vi "ziImpedanceCalibRefZ.vi"(3 "Frequencies (Hz)":dbl[](array[numeric]), 4 "Model Values":cdb[](array[numeric]), 5 "Eq Model (Unity)":T1) -> (0 "Z (Ohm)":cdb[](array[numeric]), 1 "cal_types":cluster{string[], bool[]}[](array[cluster]))   [LabVIEW 2016, in "Zurich Instruments LabOne.lvlib"]
doc: "Calculates the nominal impedance of the equivalent circuit model of the calibration reference for the frequencies used in the current measurement."
uses:
  Zurich Instruments LabOne.lvlib
  ziTypeImpedanceEqCircModel.ctl
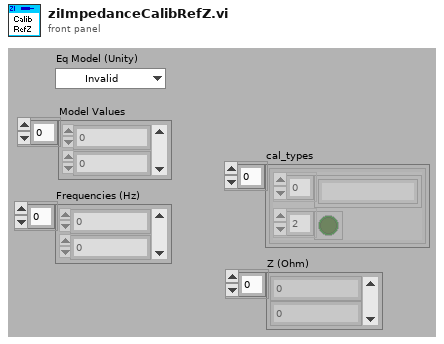
[diagram p1: front panel]
types:
  T1 = typedef "Zurich Instruments LabOne.lvlib/ziTypeImpedanceEqCircModel.ctl" = enum16{"Invalid", "|Z|, Phi", "R||C", "R||L", "R*C", "D*C", "R*L", "ReZ, ImZ", "G, B"}
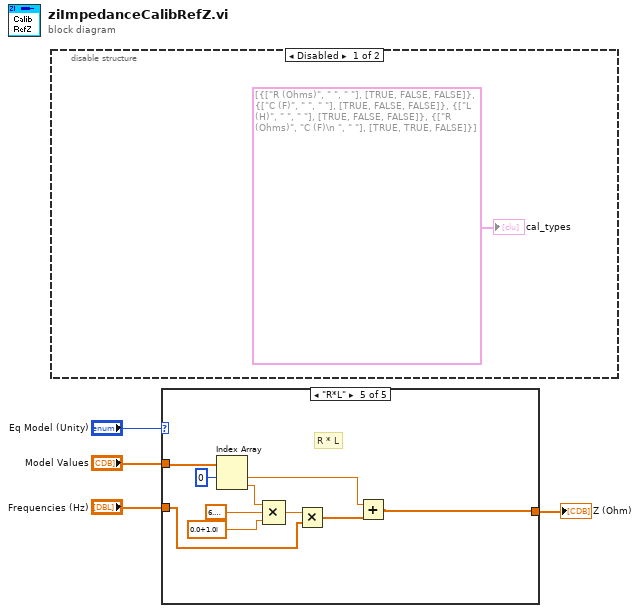
[diagram p0: block diagram]
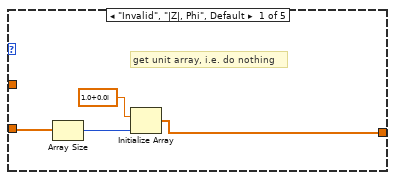
[diagram p3: hidden frame]
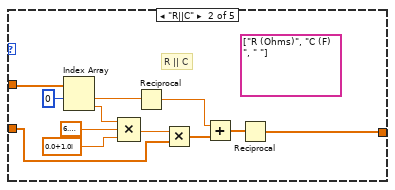
[diagram p4: hidden frame]
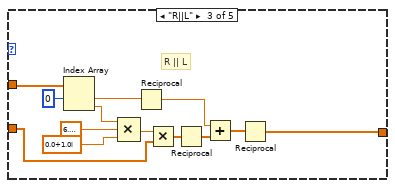
[diagram p5: hidden frame]
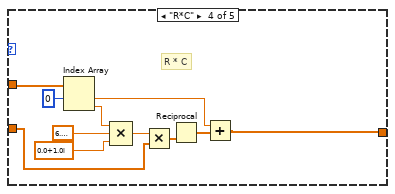
[diagram p6: hidden frame]
diagram:
  n1 = disable-structure shown="Disabled" {
    frame Disabled {
      "cal_types" <- cluster{string[], bool[]}[] [{["R (Ohms)", " ", " "], [TRUE, FALSE, FALSE]}, {["C (F)", " ", " "], [TRUE, FALSE, FALSE]}, {["L (H)", " ", " "], [TRUE, FALSE, FALSE]}, {["R (Ohms)", "C (F)\n ", " "], [TRUE, TRUE, FALSE]}]
    }
    frame Enabled {
    }
  }
  n2 = case shown="\"R*L\"" "Eq Model (Unity)" {
    tunnel: "Frequencies (Hz)" -> [w8 w11 w24 w35 w47]
    tunnel: [w6 w13 w26 w38 w49] -> w4
    tunnel: "Model Values" -> [_ w20 w33 w44 w54]
    frame "Invalid", "|Z|, Phi", Default {
      # "get unit array, i.e. do nothing"
      n3 = Array Size(array=w8) -> (size(s)=w9:i32)
      n4 = Initialize Array(cdb 1.0+0.0i, w9) -> (w6:cdb[])
    }
    frame "R||C" {
      (unwired) string[] ["R (Ohms)", "C (F) ", " "]
      # "R || C"
      n5 = Index Array(array=w20, index #1=0 ("index")) -> (element #1=w16:cdb, element #2=w17:cdb)  [unwired: 1 in]
      n6 = Compound Arithmetic op=MULTIPLY(w17, 6.283185307179586, cdb 0.0+1.0i) -> (w12:cdb)
      n7 = Reciprocal(x=w16) -> (1/x=w15:cdb)
      n8 = Multiply(x=w12, y=w11) -> (x*y=w10:cdb[])
      n9 = Add(x=w15, y=w10) -> (x+y=w14:cdb[])
      n10 = Reciprocal(x=w14) -> (1/x=w13:cdb[])
    }
    frame "R||L" {
      # "R || L"
      n11 = Index Array(array=w33, index #1=0 ("index")) -> (element #1=w29:cdb, element #2=w30:cdb)  [unwired: 1 in]
      n12 = Compound Arithmetic op=MULTIPLY(w30, 6.283185307179586, cdb 0.0+1.0i) -> (w25:cdb)
      n13 = Reciprocal(x=w29) -> (1/x=w28:cdb)
      n14 = Multiply(x=w25, y=w24) -> (x*y=w23:cdb[])
      n15 = Reciprocal(x=w23) -> (1/x=w22:cdb[])
      n16 = Add(x=w28, y=w22) -> (x+y=w27:cdb[])
      n17 = Reciprocal(x=w27) -> (1/x=w26:cdb[])
    }
    frame "R*C" {
      # "R * C"
      n18 = Index Array(array=w44, index #1=0 ("index")) -> (element #1=w37:cdb, element #2=w41:cdb)  [unwired: 1 in]
      n19 = Compound Arithmetic op=MULTIPLY(w41, 6.283185307179586, cdb 0.0+1.0i) -> (w40:cdb)
      n20 = Multiply(x=w40, y=w35) -> (x*y=w36:cdb[])
      n21 = Reciprocal(x=w36) -> (1/x=w39:cdb[])
      n22 = Add(x=w37, y=w39) -> (x+y=w38:cdb[])
    }
    frame "R*L" {
      # "R * L"
      n23 = Index Array(array=w54, index #1=0 ("index")) -> (element #1=w48:cdb, element #2=w51:cdb)  [unwired: 1 in]
      n24 = Compound Arithmetic op=MULTIPLY(w51, 6.283185307179586, cdb 0.0+1.0i) -> (w50:cdb)
      n25 = Multiply(x=w50, y=w47) -> (x*y=w46:cdb[])
      n26 = Add(x=w48, y=w46) -> (x+y=w49:cdb[])
    }
  }
  "Z (Ohm)" <- w4
